vi "SplineHelp_GetQuinticSplinesFromWeightedWayPts.vi"(11 "WeightedWayPoints":T1[](array[typedef]) {"SCALAR" format="%14.3f"; "ROTATION"."SIN" format="%13.4f"; "ROTATION"."COS" format="%13.4f"; "ROTATION"."VALUE" format="%13.4f"; "TRANSLATION"."Y" format="%14.3f"; "TRANSLATION"."X" format="%14.3f"}) -> (0 "out Error":errorcluster, 3 "Splines":T4[](array[typedef]))   [LabVIEW 2019, in "Trajectory_Library.lvlib"]
doc: "Returns quintic splines from a set of weighted waypoints.\n\nParameters:\n - weighted waypoints - The array of weighted waypoints \n\nReturns:\n - Splines - Array of splines"
uses:
  Trajectory_Library.lvlib
  <vilib>/Analysis/Matrix/Datatypes/RealMatrix.ctl
  <vilib>/Analysis/Matrix/NI_Matrix.lvlib
  TypeDef/SPLINE.ctl
  TypeDef/TRANSLATION2D.ctl
  TypeDef/ROTATION2D.ctl
  TypeDef/WEIGHTED_WAYPOINT.ctl
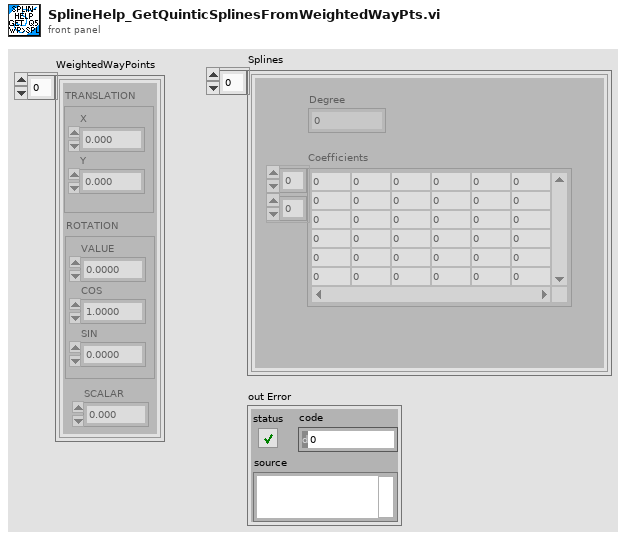
[diagram p1: front panel]
types:
  T1 = typedef "Trajectory_Library.lvlib/WEIGHTED_WAYPOINT.ctl" = cluster{"TRANSLATION":T2, "ROTATION":T3, "SCALAR":dbl}
  T2 = typedef "Trajectory_Library.lvlib/TRANSLATION2D.ctl" = cluster{"X":dbl, "Y":dbl}
  T3 = typedef "Trajectory_Library.lvlib/ROTATION2D.ctl" = cluster{"VALUE":dbl, "COS":dbl, "SIN":dbl}
  T4 = typedef "Trajectory_Library.lvlib/SPLINE.ctl" = cluster{"Degree":i32, "Coefficients":T5}
  T5 = typedef "NI_Matrix.lvlib/RealMatrix.ctl" = dbl[][]
  T6 = typedef "Trajectory_Library.lvlib/POSE2D.ctl" = cluster{"TRANSLATION":T2, "ROTATION":T3}
  T7 = typedef "Trajectory_Library.lvlib/SPLINE_CTRL_VECTOR.ctl" = cluster{"Xs":dbl[], "Ys":dbl[]}
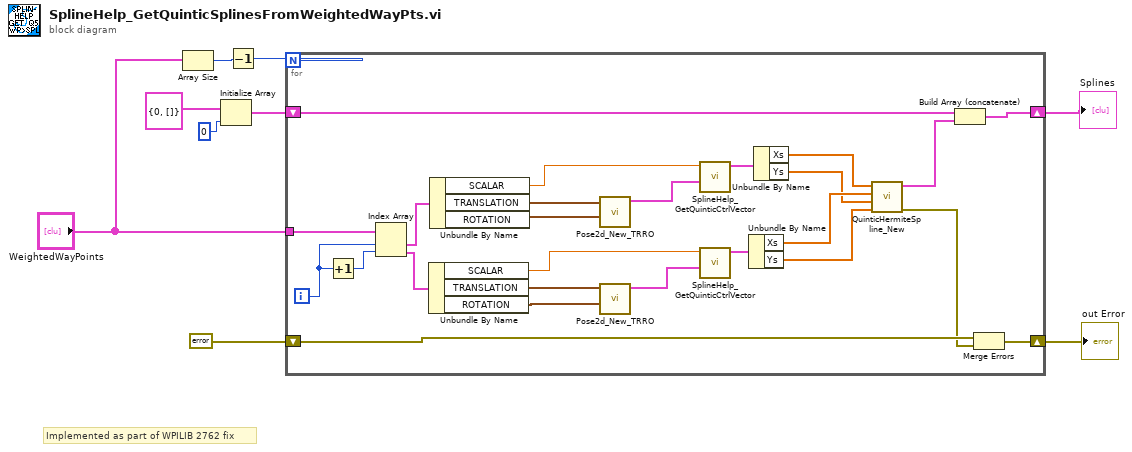
[diagram p0: block diagram]
diagram:
  # "Implemented as part of WPILIB 2762 fix"
  n1 = Array Size(array="WeightedWayPoints") -> (size(s)=w8:i32)
  n2 = Initialize Array(T4 {"Degree"=0, "Coefficients"=[]} ("SPLINE"), 0 ("dimension size")) -> (w5:T4[])
  n3 = Decrement(x=w8) -> (x-1=w9:i32)
  n4 = for {
    N: w9 -> [_]
    tunnel: "WeightedWayPoints" -> [w33]
    shift-right: [w30] -> w3
    shift-left: w5 -> [w32]
    shift-right: [w28] -> w1
    shift-left: errorcluster {"status"=FALSE, "code"=0, "source"=""} ("error constant") -> [w27]
    i -> [w31]
    n5 = Increment(x=w31) -> (x+1=w34:i32)
    n6 = Index Array(array=w33, index #1=w31, index #2=w34) -> (element #1=w18:T1, element #2=w19:T1)
    n7 = Unbundle By Name(w19) -> ("SCALAR"=w16:dbl, "TRANSLATION"=w13:T2, "ROTATION"=w12:T3)
    n8 = Unbundle By Name(w18) -> ("SCALAR"=w17:dbl, "TRANSLATION"=w11:T2, "ROTATION"=w10:T3)
    n9 = call "Pose2d_New_TRRO.vi"("ROTATION"=w10, "TRANSLATION"=w11) -> ("outPOSE"=w15:T6)  [unwired: 9 in]
    n10 = call "Pose2d_New_TRRO.vi"("ROTATION"=w12, "TRANSLATION"=w13) -> ("outPOSE"=w14:T6)  [unwired: 9 in]
    n11 = call "SplineHelp_GetQuinticCtrlVector.vi"("Input POSE"=w15, "Scalar"=w17) -> ("resultSpline_Ctrl_Vector"=w24:T7)  [unwired: 9 in]
    n12 = call "SplineHelp_GetQuinticCtrlVector.vi"("Input POSE"=w14, "Scalar"=w16) -> ("resultSpline_Ctrl_Vector"=w25:T7)  [unwired: 9 in]
    n13 = Unbundle By Name(w25) -> ("Xs"=w22:dbl[], "Ys"=w20:dbl[])
    n14 = Unbundle By Name(w24) -> ("Xs"=w23:dbl[], "Ys"=w21:dbl[])
    n15 = call "QuinticHermiteSpline_New.vi"("yFinalCtrlVector"=w20, "yInitialCtrlVector"=w21, "xFinalCtrlVector"=w22, "XInitialCtrlVector"=w23) -> ("error out"=w26:errorcluster, "QuinticHermiteSpline"=w29:T4)  [unwired: 6 in]
    n16 = Build Array (concatenate)(w32, w29) -> (w30:T4[])
    n17 = Merge Errors(w27, w26) -> (w28:errorcluster)
  }
  "Splines" <- w3
  "out Error" <- w1
